vi "sub_DC Power Start.vi"(0 "IVI引用句柄输入":refnum<k15>="Dev1" caption="Resource Name", 1 "Current Limit":dbl=0.1 format="%.3p", 3 "Voltage Level Range":dbl=6.0 format="%.5p", 4 "Current Limit Range":dbl=0.1 format="%.3p", 6 "Voltage Level":dbl=2.0 format="%.5p", 7 "Source Delay (Sec)":dbl=0.1 format="%.3p", 10 "Channel Name":string="0", 11 "Channel Name 2":string="0" caption="Channel Name", 18 "Voltage Level 2":dbl=2.0 caption="Voltage Level" format="%.5p") -> (9 "instrument handle out 2":refnum<k15>, 12 "instrument handle out":refnum<k15>, 13 "Channel Name 6":string="0" caption="Channel Name", 14 "IVI引用句柄输出":refnum<k15>, 15 "Channel Name 4":string, 17 "Channel Name 3":string, 19 "错误输出":errorcluster)   [LabVIEW 2015]
uses:
  <instrlib>/niDCPower/nidcpower.llb/niDCPower Source Mode.ctl
  <instrlib>/niDCPower/nidcpower.llb/niDCPower Output Function.ctl
  <instrlib>/niDCPower/nidcpower.llb/niDCPower Wait For Event - Event.ctl
panel:
  in  "Channel Name 5":string="0" caption="Channel Name"
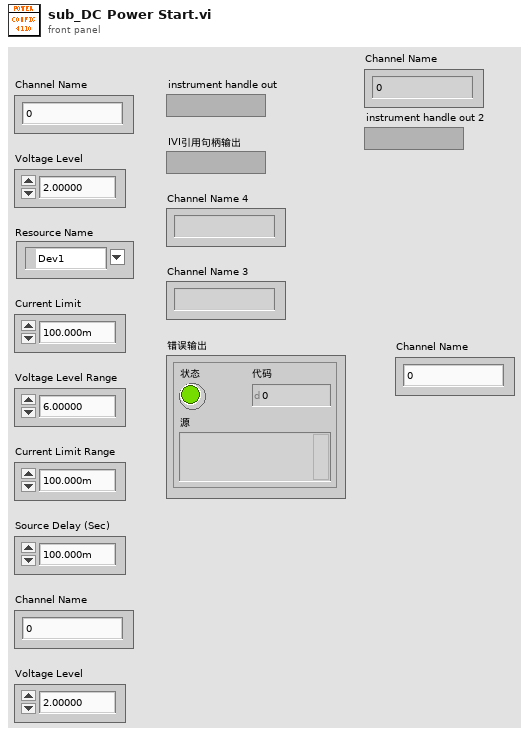
[diagram p1: front panel]
types:
  T1 = typedef "niDCPower Wait For Event - Event.ctl" = i32
  T2 = typedef "niDCPower Output Function.ctl" = i32
  T3 = typedef "niDCPower Source Mode.ctl" = i32
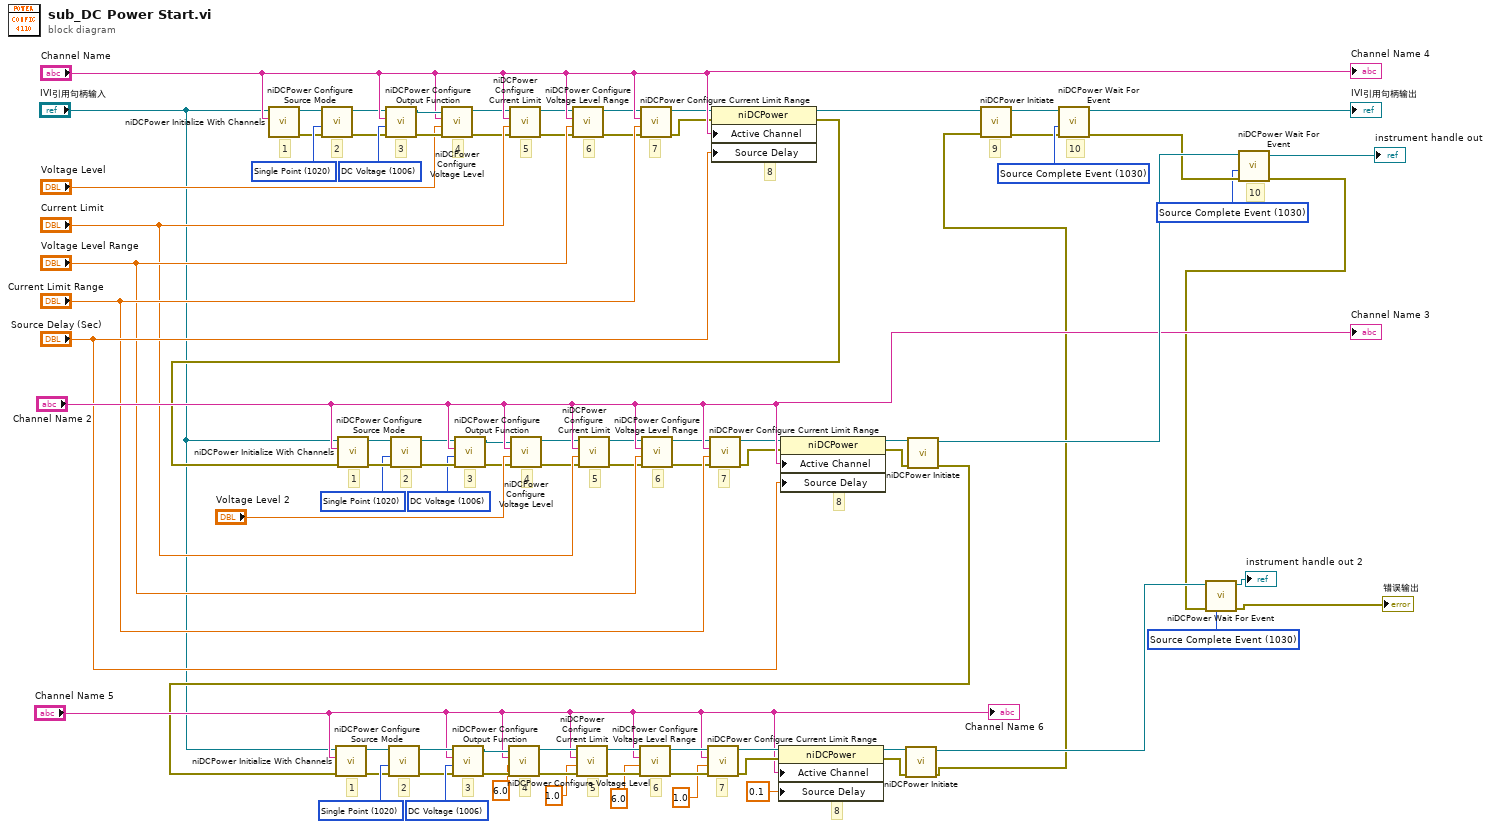
[diagram p0: block diagram]
diagram:
  w4 = T1 1030 items=["Source Complete Event"=1030, "Measure Complete Event"=1031, "Sequence Iteration Complete Event"=1032, "Sequence Engine Done Event"=1033, "Pulse Complete Event"=1051, "Ready For Pulse Trigger Event"=1052] ("event")
  w33 = T2 1006 items=["DC Voltage"=1006, "DC Current"=1007, "Pulse Voltage"=1049, "Pulse Current"=1050] ("output function")
  w24 = T3 1020 items=["Single Point"=1020, "Sequence"=1021] ("source mode")
  w82 = T1 1030 items=["Source Complete Event"=1030, "Measure Complete Event"=1031, "Sequence Iteration Complete Event"=1032, "Sequence Engine Done Event"=1033] ("event")
  w56 = T2 1006 items=["DC Voltage"=1006, "DC Current"=1007, "Pulse Voltage"=1049, "Pulse Current"=1050] ("output function")
  w65 = T3 1020 items=["Single Point"=1020, "Sequence"=1021] ("source mode")
  w55 = T2 1006 items=["DC Voltage"=1006, "DC Current"=1007, "Pulse Voltage"=1049, "Pulse Current"=1050] ("output function")
  w52 = T1 1030 items=["Source Complete Event"=1030, "Measure Complete Event"=1031, "Sequence Iteration Complete Event"=1032, "Sequence Engine Done Event"=1033] ("event")
  w41 = T3 1020 items=["Single Point"=1020, "Sequence"=1021] ("source mode")
  # "7"
  # "6"
  # "2"
  # "3"
  # "8"
  # "5"
  # "4"
  # "1"
  # "10"
  # "7"
  # "6"
  # "2"
  # "3"
  # "8"
  # "5"
  # "4"
  # "1"
  # "9"
  # "10"
  # "7"
  # "6"
  # "2"
  # "3"
  # "8"
  # "5"
  # "4"
  # "1"
  n1 = call <instrlib>:"niDCPower Initialize With Channels.vi"("channels"="Channel Name", "resource name"="IVI引用句柄输入") -> ("error out"=w37:errorcluster, "instrument handle out"=w38:refnum<k15>)  [unwired: 3 in, 5 out]
  n2 = call <instrlib>:"niDCPower Configure Source Mode.vi"("error in (no error)"=w37, "source mode"=w41, "instrument handle"=w38) -> ("error out"=w39:errorcluster, "instrument handle out"=w40:refnum<k15>)  [unwired: 7 out]
  n3 = call <instrlib>:"niDCPower Configure Output Function.vi"("error in (no error)"=w39, "output function"=w55, "channel name"="Channel Name", "instrument handle"=w40) -> ("error out"=w54:errorcluster, "instrument handle out"=w53:refnum<k15>)  [unwired: 6 out]
  n4 = call <instrlib>:"niDCPower Configure Voltage Level.vi"("error in (no error)"=w54, "voltage level"="Voltage Level", "channel name"="Channel Name", "instrument handle"=w53) -> ("error out"=w35:errorcluster, "instrument handle out"=w34:refnum<k15>)  [unwired: 6 out]
  n5 = call <instrlib>:"niDCPower Configure Current Limit.vi"("error in (no error)"=w35, "current limit"="Current Limit", "channel name"="Channel Name", "instrument handle"=w34) -> ("error out"=w42:errorcluster, "instrument handle out"=w43:refnum<k15>)  [unwired: 1 in, 5 out]
  n6 = call <instrlib>:"niDCPower Configure Voltage Level Range.vi"("error in (no error)"=w42, "voltage level range"="Voltage Level Range", "channel name"="Channel Name", "instrument handle"=w43) -> ("error out"=w44:errorcluster, "instrument handle out"=w45:refnum<k15>)  [unwired: 6 out]
  n7 = call <instrlib>:"niDCPower Configure Current Limit Range.vi"("error in (no error)"=w44, "current limit range"="Current Limit Range", "channel name"="Channel Name", "instrument handle"=w45) -> ("error out"=w47:errorcluster, "instrument handle out"=w46:refnum<k15>)  [unwired: 6 out]
  n8 = property class="niDCPower"(reference=w46, error in=w47, "Active Channel"="Channel Name", "Source Delay"="Source Delay (Sec)") -> (reference out=w73:refnum<k15>, error out=w74:errorcluster)
  n9 = call <instrlib>:"niDCPower Initialize With Channels.vi"("error in (no error)"=w74, "channels"="Channel Name 2", "resource name"="IVI引用句柄输入") -> ("error out"=w69:errorcluster, "instrument handle out"=w68:refnum<k15>)  [unwired: 2 in, 5 out]
  n10 = call <instrlib>:"niDCPower Configure Source Mode.vi"("error in (no error)"=w69, "source mode"=w65, "instrument handle"=w68) -> ("error out"=w67:errorcluster, "instrument handle out"=w66:refnum<k15>)  [unwired: 7 out]
  n11 = call <instrlib>:"niDCPower Configure Output Function.vi"("error in (no error)"=w67, "output function"=w56, "channel name"="Channel Name 2", "instrument handle"=w66) -> ("error out"=w57:errorcluster, "instrument handle out"=w58:refnum<k15>)  [unwired: 6 out]
  n12 = call <instrlib>:"niDCPower Configure Voltage Level.vi"("error in (no error)"=w57, "voltage level"="Voltage Level 2", "channel name"="Channel Name 2", "instrument handle"=w58) -> ("error out"=w71:errorcluster, "instrument handle out"=w72:refnum<k15>)  [unwired: 6 out]
  n13 = call <instrlib>:"niDCPower Configure Current Limit.vi"("error in (no error)"=w71, "current limit"="Current Limit", "channel name"="Channel Name 2", "instrument handle"=w72) -> ("error out"=w64:errorcluster, "instrument handle out"=w63:refnum<k15>)  [unwired: 1 in, 5 out]
  n14 = call <instrlib>:"niDCPower Configure Voltage Level Range.vi"("error in (no error)"=w64, "voltage level range"="Voltage Level Range", "channel name"="Channel Name 2", "instrument handle"=w63) -> ("error out"=w62:errorcluster, "instrument handle out"=w61:refnum<k15>)  [unwired: 6 out]
  n15 = call <instrlib>:"niDCPower Configure Current Limit Range.vi"("error in (no error)"=w62, "current limit range"="Current Limit Range", "channel name"="Channel Name 2", "instrument handle"=w61) -> ("error out"=w59:errorcluster, "instrument handle out"=w60:refnum<k15>)  [unwired: 6 out]
  n16 = property class="niDCPower"(reference=w60, error in=w59, "Active Channel"="Channel Name 2", "Source Delay"="Source Delay (Sec)") -> (reference out=w79:refnum<k15>, error out=w80:errorcluster)
  n17 = call <instrlib>:"niDCPower Initiate.vi"("error in (no error)"=w80, "instrument handle"=w79) -> ("error out"=w14:errorcluster, "instrument handle out"=w84:refnum<k15>)  [unwired: 2 in, 6 out]
  n18 = call <instrlib>:"niDCPower Initialize With Channels.vi"("error in (no error)"=w14, "channels"="Channel Name 5", "resource name"="IVI引用句柄输入") -> ("error out"=w20:errorcluster, "instrument handle out"=w21:refnum<k15>)  [unwired: 2 in, 5 out]
  n19 = call <instrlib>:"niDCPower Configure Source Mode.vi"("error in (no error)"=w20, "source mode"=w24, "instrument handle"=w21) -> ("error out"=w22:errorcluster, "instrument handle out"=w23:refnum<k15>)  [unwired: 7 out]
  n20 = call <instrlib>:"niDCPower Configure Output Function.vi"("error in (no error)"=w22, "output function"=w33, "channel name"="Channel Name 5", "instrument handle"=w23) -> ("error out"=w32:errorcluster, "instrument handle out"=w31:refnum<k15>)  [unwired: 6 out]
  n21 = call <instrlib>:"niDCPower Configure Voltage Level.vi"("error in (no error)"=w32, "voltage level"=6.0, "channel name"="Channel Name 5", "instrument handle"=w31) -> ("error out"=w19:errorcluster, "instrument handle out"=w18:refnum<k15>)  [unwired: 6 out]
  n22 = call <instrlib>:"niDCPower Configure Current Limit.vi"("error in (no error)"=w19, "current limit"=1.0, "channel name"="Channel Name 5", "instrument handle"=w18) -> ("error out"=w25:errorcluster, "instrument handle out"=w26:refnum<k15>)  [unwired: 1 in, 5 out]
  n23 = call <instrlib>:"niDCPower Configure Voltage Level Range.vi"("error in (no error)"=w25, "voltage level range"=6.0, "channel name"="Channel Name 5", "instrument handle"=w26) -> ("error out"=w27:errorcluster, "instrument handle out"=w28:refnum<k15>)  [unwired: 6 out]
  n24 = call <instrlib>:"niDCPower Configure Current Limit Range.vi"("error in (no error)"=w27, "current limit range"=1.0, "channel name"="Channel Name 5", "instrument handle"=w28) -> ("error out"=w30:errorcluster, "instrument handle out"=w29:refnum<k15>)  [unwired: 6 out]
  n25 = property class="niDCPower"(reference=w29, error in=w30, "Active Channel"="Channel Name 5", "Source Delay"=0.1 ("Source:Advanced:Source Delay")) -> (reference out=w17:refnum<k15>, error out=w16:errorcluster)
  n26 = call <instrlib>:"niDCPower Initiate.vi"("error in (no error)"=w16, "instrument handle"=w17) -> ("error out"=w9:errorcluster, "instrument handle out"=w10:refnum<k15>)  [unwired: 2 in, 6 out]
  n27 = call <instrlib>:"niDCPower Initiate.vi"("error in (no error)"=w9, "instrument handle"=w73) -> ("error out"=w51:errorcluster, "instrument handle out"=w49:refnum<k15>)  [unwired: 2 in, 6 out]
  n28 = call <instrlib>:"niDCPower Wait For Event.vi"("error in (no error)"=w51, "event"=w52, "instrument handle"=w49) -> ("error out"=w83:errorcluster, "instrument handle out"=→"IVI引用句柄输出":refnum<k15>)  [unwired: 1 in, 6 out]
  n29 = call <instrlib>:"niDCPower Wait For Event.vi"("error in (no error)"=w83, "event"=w82, "instrument handle"=w84) -> ("error out"=w6:errorcluster, "instrument handle out"=→"instrument handle out":refnum<k15>)  [unwired: 1 in, 6 out]
  n30 = call <instrlib>:"niDCPower Wait For Event.vi"("error in (no error)"=w6, "event"=w4, "instrument handle"=w10) -> ("error out"=→"错误输出":errorcluster, "instrument handle out"=→"instrument handle out 2":refnum<k15>)  [unwired: 1 in, 6 out]
  "Channel Name 3" <- "Channel Name 2"
  "Channel Name 4" <- "Channel Name"
  "Channel Name 6" <- "Channel Name 5"
